vi "Create Py Object Int32.vi"(8 "error in (no error)":errorcluster, 10 "Value":i32, 11 "Session Handle in":refnum<data-value>) -> (0 "error out":errorcluster, 2 "Python Object Refnum":T1, 3 "Session Handle out":refnum<data-value>)   [LabVIEW 2020, in "G-Embedded-Python-Interpreter-Toolkit.lvlib"]
uses:
  G-Embedded-Python-Interpreter-Toolkit.lvlib
  Python Object Reference.ctl
  Python Object Type.ctl
  bin/gepit.cp310.32.dll
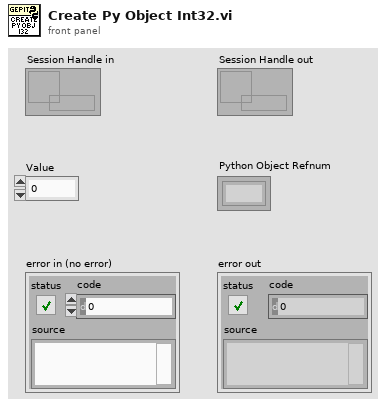
[diagram p1: front panel]
types:
  T1 = typedef "G-Embedded-Python-Interpreter-Toolkit.lvlib/Python Object Reference.ctl" = refnum<k1>
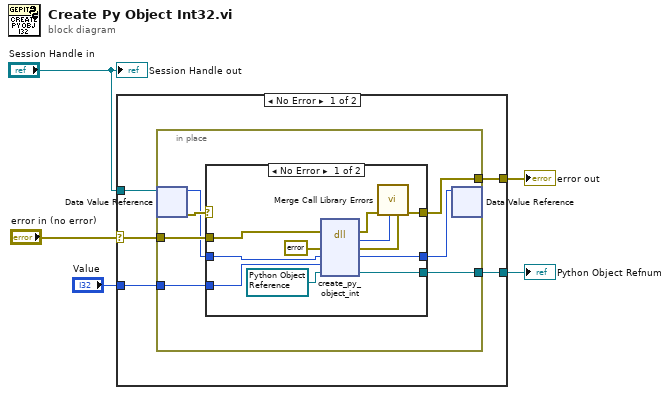
[diagram p0: block diagram]
diagram:
  n1 = case shown="No Error" "error in (no error)" {
    selector: "error in (no error)" -> [w9 w31]
    tunnel: "Session Handle in" -> [w10 _]
    tunnel: [w8 w31] -> w4
    tunnel: [w7 _] -> w2
    tunnel: "Value" -> [w6 _]
    frame No Error {
      n2 = in-place {
        in-place-border: w9 -> [w16]
        in-place-border: [w13] -> w8
        in-place-border: [w12] -> w7
        in-place-border: w6 -> [w11]
        n3 = in-place-dvr #1(w10) -> (w15:u64, w17:errorcluster)
        n4 = case shown="No Error" w17 {
          selector: w17 -> [_ w29]
          tunnel: w16 -> [w24 _]
          tunnel: w15 -> [w23 w30]
          tunnel: [w22 w30] -> w14
          tunnel: [w21 w29] -> w13
          tunnel: [w20 _] -> w12
          tunnel: w11 -> [w18 _]
          frame No Error {
            w19 = T1 refnum items=["PObj"] ("Py Object")
            n5 = dll-call lib="C:/serenial/libraries/g-embedded-python-interpreter-toolkit/LabVIEW/bin/gepit.cp310.32.dll" fn="create_py_object_int"(error in=w24, "Error"=errorcluster {"status"=FALSE, "code"=0, "source"=""} ("error constant"), "Session"=w23, "Value"=w18, "Py Object"=w19) -> (error out=w27:errorcluster, "return type"=w26:i32, "Error"=w25:errorcluster, "Session"=w22:u64, "Py Object"=w20:T1)  [unwired: 3 in, 1 out]
            n6 = call "Merge Call Library Errors.vi"("Call Library Error"=w25, "Return Value"=w26, "error in"=w27) -> ("error out"=w21:errorcluster)  [unwired: 8 in]
          }
          frame Error {
          }
        }
        n7 = in-place-dvr #1(w14) -> ()  [unwired: 2 out]
      }
    }
    frame Error {
    }
  }
  "error out" <- w4
  "Python Object Refnum" <- w2
  "Session Handle out" <- "Session Handle in"
